vi "h10 do it yrself.vi"() -> ()   [LabVIEW 2017]
panel:
  out "stop":bool
  out "tijd":dbl
  out "Boolean":bool
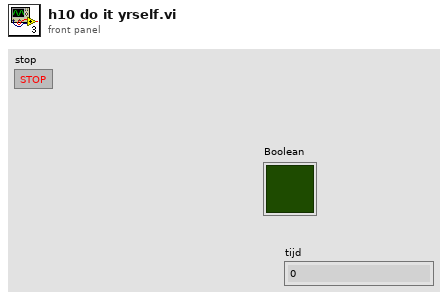
[diagram p1: front panel]
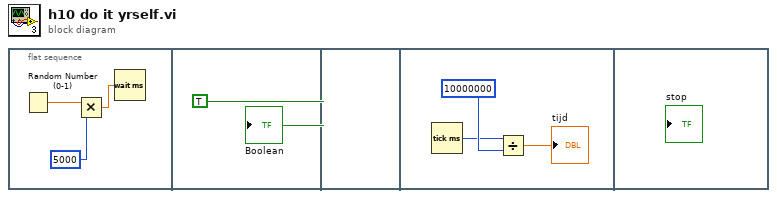
[diagram p0: block diagram]
diagram:
  n1 = flat-sequence {
    frame #0 {
      n2 = Random Number (0-1)() -> (number: 0 to 1=w2:dbl)
      n3 = Multiply(x=w2, y=5000) -> (x*y=w1:dbl)
      n4 = Wait (ms)(milliseconds to wait=w1) -> ()  [unwired: 1 out]
    }
    frame #1 {
      "Boolean" <- TRUE
    }
    frame #2 {
    }
    frame #3 {
      n5 = Tick Count (ms)() -> (millisecond timer value=w6:u32)
      n6 = Divide(x=w6, y=10000000) -> (x/y=→"tijd":dbl)
    }
    frame #4 {
    }
  }
